vi "sensor cmd debug get.vi"(9 "data":u32, 10 "id":u8, 11 "device_handle":u32) -> (1 "data out":u32, 2 "function return":i32, 3 "device_handle out":u32)   [LabVIEW 2019, in "apdm.lvlib"]
doc: "APDM_EXPORT int apdm_sensor_cmd_debug_get(apdm_device_handle_t device_handle, uint8_t id, uint32_t *data);"
uses:
  apdm.lvlib
  Lee Lab/CP FES Walking 2018/Code/Working/LabVIEW/apdm.dll
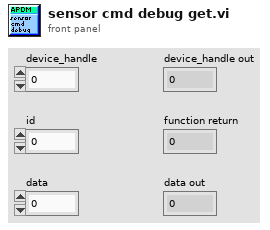
[diagram p1: front panel]
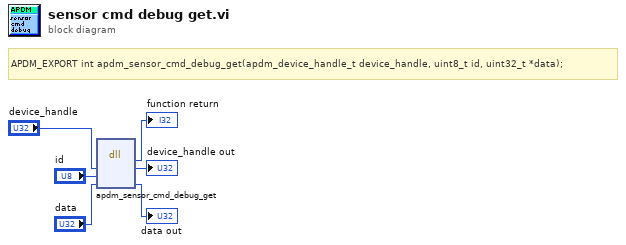
[diagram p0: block diagram]
diagram:
  # "APDM_EXPORT int apdm_sensor_cmd_debug_get(apdm_device_handle_t device_handle, uint8_t id, uint32_t *data);"
  n1 = dll-call lib="C:/Users/jfalesi/Dropbox/Lee Lab/CP FES Walking 2018/Code/Working/LabVIEW/apdm.*" fn="apdm_sensor_cmd_debug_get"("device_handle"="device_handle", "id"="id", "data"="data") -> (→"function return":i32, "device_handle"=→"device_handle out":u32, "data"=→"data out":u32)  [unwired: 4 in, 2 out]
